vi "CRYSet curve select Front Panel.vi"(11 "Vi Ref":refnum<vi>) -> ()   [LabVIEW 2013]
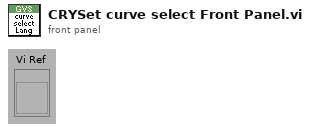
[diagram p1: front panel]
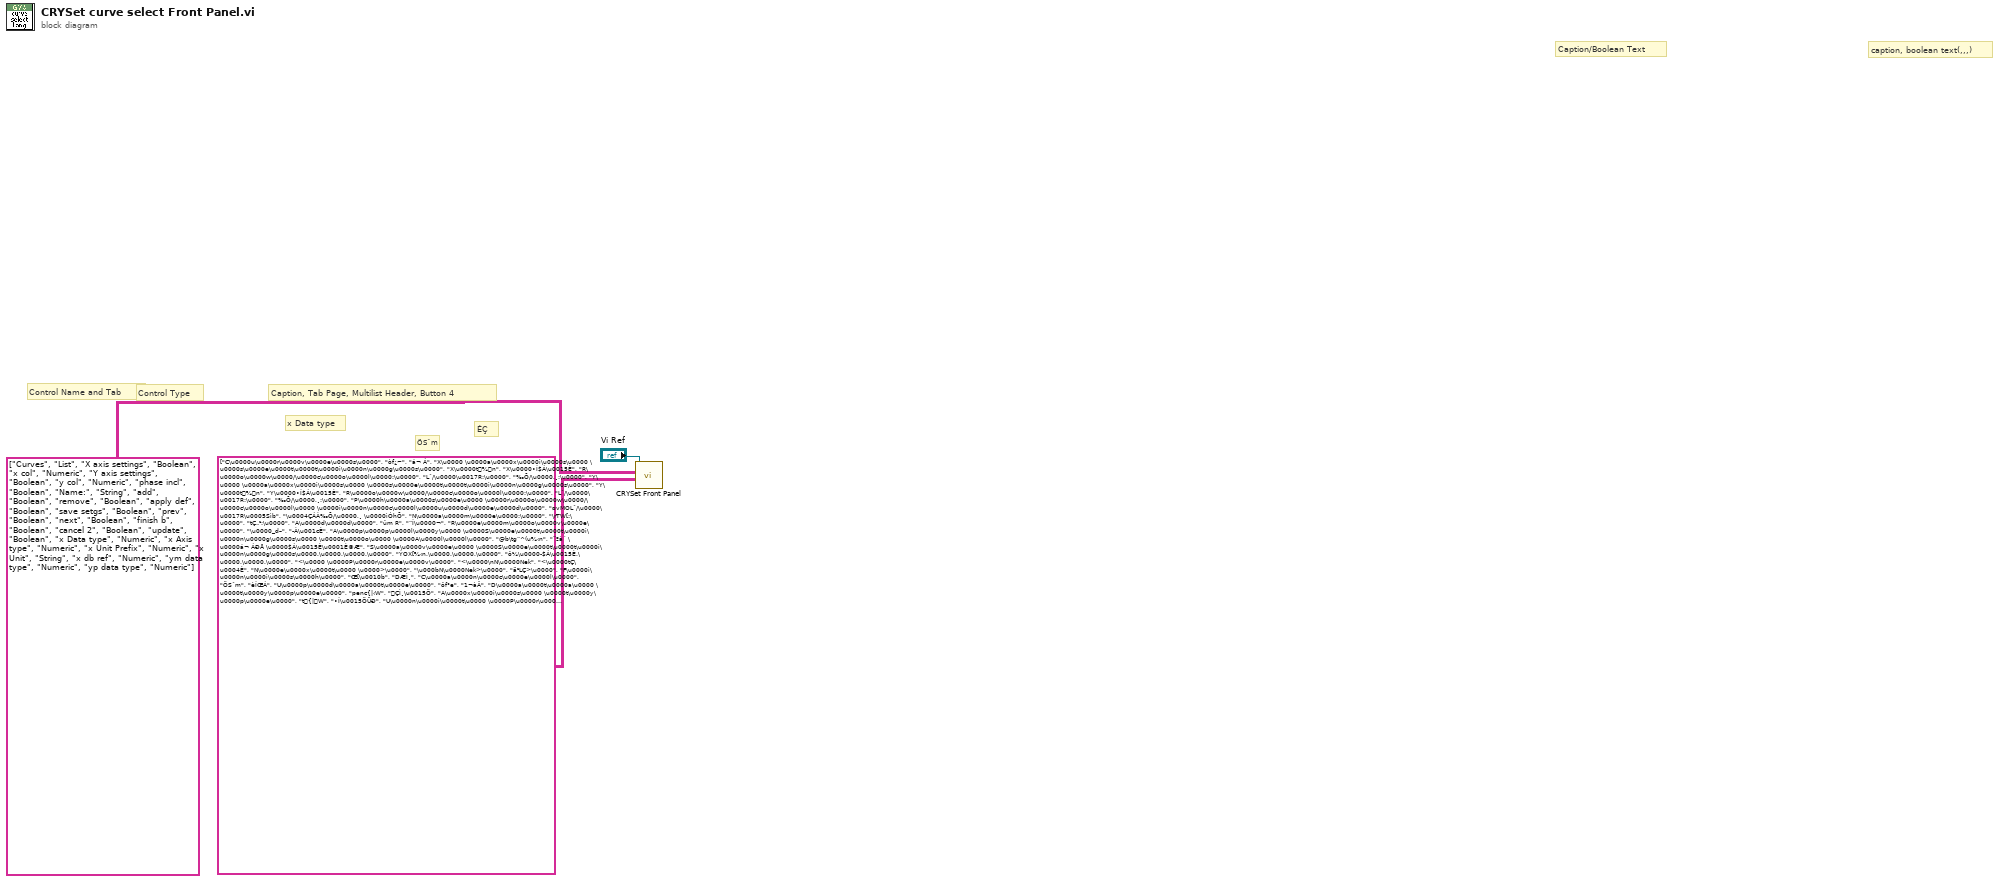
[diagram p0: block diagram]
diagram:
  # "ÉÇ"
  # "ÖSˆm"
  # "x Data type"
  # "Caption, Tab Page, Multilist Header, Button 4"
  # "Control Type"
  # "Control Name and Tab"
  # "caption, boolean text(,,,)"
  # "Caption/Boolean Text"
  n1 = call "CRYSet Front Panel.vi"("Caption(Boolean Text)"=string[][] [["C\u0000u\u0000r\u0000v\u0000e\u0000s\u0000", "òf¿~", "á¬ Á"], ["X\u0000 \u0000a\u0000x\u0000i\u0000s\u0000 \u0000s\u0000e\u0000t\u0000t\u0000i\u0000n\u0000g\u0000s\u0000", "X\u0000t¾n", "X\u0000•Í$Á\u0015È"], ["R\u0000o\u0000w\u0000/\u0000c\u0000o\u0000l\u0000:\u0000", "Lˆ/\u0000\u0017R:\u0000", "‰Õ/\u0000,¸:\u0000"], ["Y\u0000 \u0000a\u0000x\u0000i\u0000s\u0000 \u0000s\u0000e\u0000t\u0000t\u0000i\u0000n\u0000g\u0000s\u0000", "Y\u0000t¾n", "Y\u0000•Í$Á\u0015È"], ["R\u0000o\u0000w\u0000/\u0000c\u0000o\u0000l\u0000:\u0000", "Lˆ/\u0000\u0017R:\u0000", "‰Õ/\u0000,¸:\u0000"], ["P\u0000h\u0000a\u0000s\u0000e\u0000 \u0000r\u0000o\u0000w\u0000/\u0000c\u0000o\u0000l\u0000 \u0000i\u0000n\u0000c\u0000l\u0000u\u0000d\u0000e\u0000d\u0000", "øvMOLˆ/\u0000\u0017R\u0005Sìb", "\u0004ÇÁÀ‰Õ/\u0000,¸ \u0000ìÓhÕ"], ["N\u0000a\u0000m\u0000e\u0000:\u0000", "\rTW[:\u0000", "tÇ„¹:\u0000"], ["A\u0000d\u0000d\u0000", "ûm R", "”Í\u0000¬"], ["R\u0000e\u0000m\u0000o\u0000v\u0000e\u0000", "\u0000_d–", "­À\u001cÈ"], ["A\u0000p\u0000p\u0000l\u0000y\u0000 \u0000S\u0000e\u0000t\u0000t\u0000i\u0000n\u0000g\u0000s\u0000 \u0000t\u0000o\u0000 \u0000A\u0000l\u0000l\u0000", "@b\tg”^(u¾‹n", "¨ºà´ \u0000á¬ ÁÐÅ \u0000$Á\u0015È\u0001È©Æ"], ["S\u0000a\u0000v\u0000e\u0000 \u0000S\u0000e\u0000t\u0000t\u0000i\u0000n\u0000g\u0000s\u0000.\u0000.\u0000.\u0000", "ÝOX[¾‹n.\u0000.\u0000.\u0000", "ô¼\u0000­$Á\u0015È.\u0000.\u0000.\u0000"], ["<\u0000 \u0000P\u0000r\u0000e\u0000v\u0000", "<\u0000\nN\u0000Nek", "<\u0000tÇ\u0004È"], ["N\u0000e\u0000x\u0000t\u0000 \u0000>\u0000", "\u000bN\u0000Nek>\u0000", "ä²LÇ>\u0000"], ["F\u0000i\u0000n\u0000i\u0000s\u0000h\u0000", "Œ[\u0010b", "DÆÌ¸"], ["C\u0000a\u0000n\u0000c\u0000e\u0000l\u0000", "ÖSˆm", "èÍŒÁ"], ["U\u0000p\u0000d\u0000a\u0000t\u0000e\u0000", "ôf°e", "1¬àÂ"], ["D\u0000a\u0000t\u0000a\u0000 \u0000t\u0000y\u0000p\u0000e\u0000", "penc{|‹W", "ÇÌ¸\u0015Ö"], ["A\u0000x\u0000i\u0000s\u0000 \u0000t\u0000y\u0000p\u0000e\u0000", "t{|W", "•Í\u0015ÖÜÐ"], ["U\u0000n\u0000i\u0000t\u0000 \u0000P\u0000r\u0000e\u0000f\u0000i\u0000x\u0000", "USMOMR\u0000", "è²\u0004Ç^Å™½tÇ"], ["U\u0000n\u0000i\u0000t\u0000", "USMO", "è²\u0004Ç"], ["d\u0000b\u0000 \u0000r\u0000e\u0000f\u0000.\u0000 \u0000l\u0000e\u0000v\u0000e\u0000l\u0000", "d\u0000b\u0000 \u0000r\u0000e\u0000f\u0000 \u00004ls^", "d\u0000b\u0000 \u0000r\u0000e\u0000f\u0000 \u0000\u0000É\u0004Ç"], ["M\u0000a\u0000g\u0000.\u0000", "'Y\u000f\\", "ÄÉíÓ"], ["P\u0000h\u0000a\u0000s\u0000e\u0000", "øv", "\u0004ÇÁÀ"]], "Control ID and Type(Label Name, Type)"=string[][] [["Curves", "List"], ["X axis settings", "Boolean"], ["x col", "Numeric"], ["Y axis settings", "Boolean"], ["y col", "Numeric"], ["phase incl", "Boolean"], ["Name:", "String"], ["add", "Boolean"], ["remove", "Boolean"], ["apply def", "Boolean"], ["save setgs", "Boolean"], ["prev", "Boolean"], ["next", "Boolean"], ["finish b", "Boolean"], ["cancel 2", "Boolean"], ["update", "Boolean"], ["x Data type", "Numeric"], ["x Axis type", "Numeric"], ["x Unit Prefix", "Numeric"], ["x Unit", "String"], ["x db ref", "Numeric"], ["ym data type", "Numeric"], ["yp data type", "Numeric"]], "Vi Ref"="Vi Ref") -> ()  [unwired: 9 in]
